vi "VisionNetwork.vi"(8 "error in (no error)":errorcluster) -> (0 "error out":errorcluster)   [LabVIEW 2023]
doc: "Vision Network\n\nInput\n --Error in \n\nOutput\n --Error out"
uses:
  <vilib>/Rock Robotics/WPI/ThirdParty/JAS_Junk/TrajLib/Trajectory_Library.lvlib
  <vilib>/Rock Robotics/Network Tables/NT Write Number.vi
  <vilib>/Rock Robotics/Network Tables/NT Write Boolean.vi
  <vilib>/Rock Robotics/Network Tables/NT Read Number.vi
  Vision/VisionGlobal.vi
  VisionNetworkingGlobal.vi
  <vilib>/Rock Robotics/Network Tables/NT Write Integer.vi
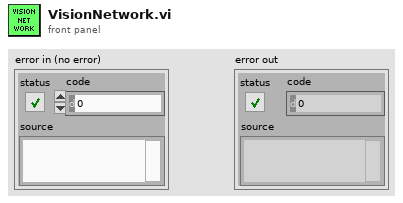
[diagram p1: front panel]
types:
  T1 = typedef "Trajectory_Library.lvlib/POSE2D.ctl" = cluster{"TRANSLATION":T2, "ROTATION":T3}
  T2 = typedef "Trajectory_Library.lvlib/TRANSLATION2D.ctl" = cluster{"X":dbl, "Y":dbl}
  T3 = typedef "Trajectory_Library.lvlib/ROTATION2D.ctl" = cluster{"VALUE":dbl, "COS":dbl, "SIN":dbl}
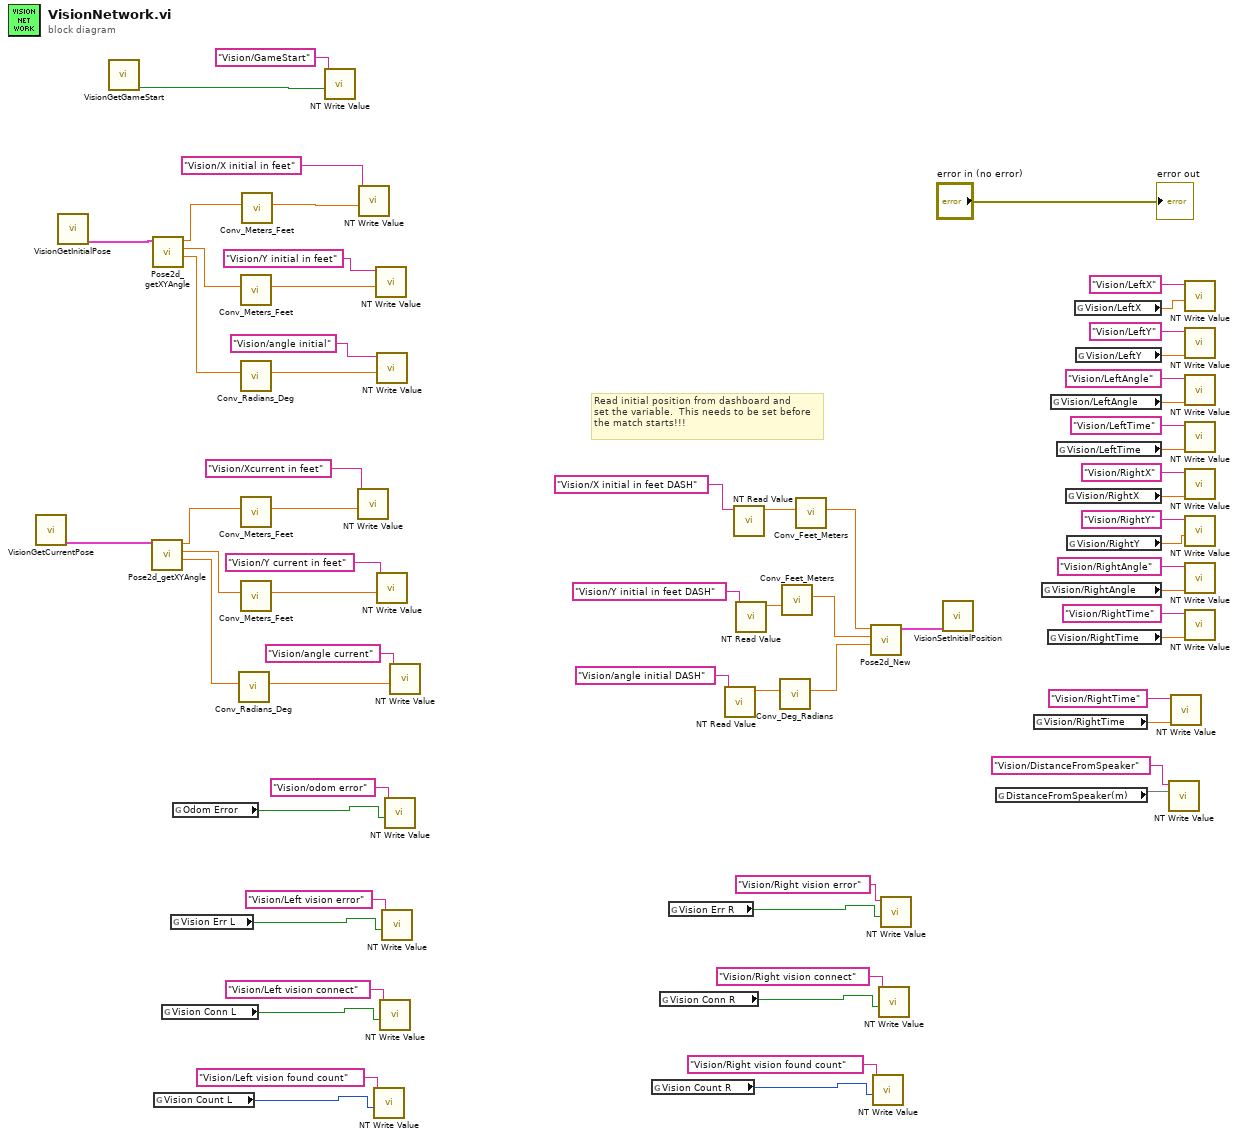
[diagram p0: block diagram]
diagram:
  # "Read initial position from dashboard and\nset the variable.  This needs to be set before\nthe match starts!!!"
  n1 = call "VisionGetCurrentPose.vi"() -> ("Current Pose"=w66:T1)  [unwired: 9 in]
  n2 = call "VisionGetInitialPose.vi"() -> ("InitialPose"=w53:T1)  [unwired: 10 in]
  n3 = call "VisionGetGameStart.vi"() -> ("Game Start"=w52:bool)  [unwired: 11 in]
  n4 = call <vilib>:"Pose2d_getXYAngle.vi"("in POSE"=w66) -> ("Angle"=w65:dbl, "Y"=w64:dbl, "X"=w63:dbl)  [unwired: 8 in]
  n5 = call <vilib>:"Pose2d_getXYAngle.vi"("in POSE"=w53) -> ("Angle"=w59:dbl, "Y"=w58:dbl, "X"=w57:dbl)  [unwired: 8 in]
  n6 = global read "VisionGlobal.vi" "Vision Count L"() -> (w27:i32)
  n7 = global read "VisionGlobal.vi" "Vision Conn L"() -> (w29:bool)
  n8 = global read "VisionGlobal.vi" "Vision Err L"() -> (w31:bool)
  n9 = global read "VisionGlobal.vi" "Odom Error"() -> (w33:bool)
  n10 = call <vilib>:"Conv_Radians_Deg.vi"("Radians"=w65) -> ("Degrees"=w60:dbl)  [unwired: 10 in]
  n11 = call <vilib>:"Conv_Meters_Feet.vi"("Meters"=w58) -> ("Feet"=w55:dbl)  [unwired: 10 in]
  n12 = call <vilib>:"Conv_Radians_Deg.vi"("Radians"=w59) -> ("Degrees"=w54:dbl)  [unwired: 10 in]
  n13 = call <vilib>:"Conv_Meters_Feet.vi"("Meters"=w63) -> ("Feet"=w62:dbl)  [unwired: 10 in]
  n14 = call <vilib>:"Conv_Meters_Feet.vi"("Meters"=w64) -> ("Feet"=w61:dbl)  [unwired: 10 in]
  n15 = call <vilib>:"Conv_Meters_Feet.vi"("Meters"=w57) -> ("Feet"=w56:dbl)  [unwired: 10 in]
  n16 = call-poly <vilib>:"NT Write Value.vi"("value"=w52, "name"="Vision/GameStart") -> ()  [unwired: 9 in, 1 out]
  n17 = call-poly <vilib>:"NT Write Value.vi"("value"=w62, "name"="Vision/Xcurrent in feet") -> ()  [unwired: 9 in, 1 out]
  n18 = call-poly <vilib>:"NT Write Value.vi"("value"=w56, "name"="Vision/X initial in feet") -> ()  [unwired: 9 in, 1 out]
  n19 = call-poly <vilib>:"NT Write Value.vi"("value"=w27, "name"="Vision/Left vision found count") -> ()  [unwired: 9 in, 1 out]
  n20 = call-poly <vilib>:"NT Write Value.vi"("value"=w55, "name"="Vision/Y initial in feet") -> ()  [unwired: 9 in, 1 out]
  n21 = call-poly <vilib>:"NT Write Value.vi"("value"=w54, "name"="Vision/angle initial") -> ()  [unwired: 9 in, 1 out]
  n22 = call-poly <vilib>:"NT Write Value.vi"("value"=w61, "name"="Vision/Y current in feet") -> ()  [unwired: 9 in, 1 out]
  n23 = call-poly <vilib>:"NT Write Value.vi"("value"=w29, "name"="Vision/Left vision connect") -> ()  [unwired: 9 in, 1 out]
  n24 = call-poly <vilib>:"NT Write Value.vi"("value"=w31, "name"="Vision/Left vision error") -> ()  [unwired: 9 in, 1 out]
  n25 = call-poly <vilib>:"NT Write Value.vi"("value"=w33, "name"="Vision/odom error") -> ()  [unwired: 9 in, 1 out]
  n26 = call-poly <vilib>:"NT Write Value.vi"("value"=w60, "name"="Vision/angle current") -> ()  [unwired: 9 in, 1 out]
  n27 = global read "VisionGlobal.vi" "Vision Count R"() -> (w22:i32)
  n28 = global read "VisionGlobal.vi" "Vision Conn R"() -> (w24:bool)
  n29 = global read "VisionGlobal.vi" "Vision Err R"() -> (w26:bool)
  n30 = call-poly <vilib>:"NT Read Value.vi"("name"="Vision/angle initial DASH") -> ("value"=w39:dbl)  [unwired: 8 in, 2 out]
  n31 = call-poly <vilib>:"NT Read Value.vi"("name"="Vision/X initial in feet DASH") -> ("value"=w42:dbl)  [unwired: 8 in, 2 out]
  n32 = call-poly <vilib>:"NT Read Value.vi"("name"="Vision/Y initial in feet DASH") -> ("value"=w41:dbl)  [unwired: 8 in, 2 out]
  n33 = call <vilib>:"Conv_Deg_Radians.vi"("Degress"=w39) -> ("Radians"=w38:dbl)  [unwired: 10 in]
  n34 = call <vilib>:"Conv_Feet_Meters.vi"("Feet"=w41) -> ("Meters"=w40:dbl)  [unwired: 10 in]
  n35 = call <vilib>:"Conv_Feet_Meters.vi"("Feet"=w42) -> ("Meters"=w43:dbl)  [unwired: 10 in]
  n36 = call <vilib>:"Pose2d_New.vi"("Heading"=w38, "Y"=w40, "X"=w43) -> ("out POSe"=w44:T1)  [unwired: 8 in]
  n37 = call-poly <vilib>:"NT Write Value.vi"("value"=w22, "name"="Vision/Right vision found count") -> ()  [unwired: 9 in, 1 out]
  n38 = call-poly <vilib>:"NT Write Value.vi"("value"=w24, "name"="Vision/Right vision connect") -> ()  [unwired: 9 in, 1 out]
  n39 = call-poly <vilib>:"NT Write Value.vi"("value"=w26, "name"="Vision/Right vision error") -> ()  [unwired: 9 in, 1 out]
  n40 = call "VisionSetInitialPosition.vi"("InitialPose"=w44) -> ()  [unwired: 11 in]
  n41 = global read "VisionGlobal.vi" "DistanceFromSpeaker(m)"() -> (w2)
  n42 = global read "VisionNetworkingGlobal.vi" "Vision/RightTime"() -> (w3:dbl)
  n43 = global read "VisionNetworkingGlobal.vi" "Vision/RightAngle"() -> (w7:dbl)
  n44 = global read "VisionNetworkingGlobal.vi" "Vision/RightTime"() -> (w5:dbl)
  n45 = global read "VisionNetworkingGlobal.vi" "Vision/LeftAngle"() -> (w15:dbl)
  n46 = global read "VisionNetworkingGlobal.vi" "Vision/LeftTime"() -> (w13:dbl)
  n47 = global read "VisionNetworkingGlobal.vi" "Vision/RightX"() -> (w11:dbl)
  n48 = global read "VisionNetworkingGlobal.vi" "Vision/RightY"() -> (w9:dbl)
  n49 = global read "VisionNetworkingGlobal.vi" "Vision/LeftX"() -> (w19:dbl)
  n50 = global read "VisionNetworkingGlobal.vi" "Vision/LeftY"() -> (w17:dbl)
  n51 = call-poly <vilib>:"NT Write Value.vi"("value"=w2, "name"="Vision/DistanceFromSpeaker") -> ()  [unwired: 9 in, 1 out]
  n52 = call-poly <vilib>:"NT Write Value.vi"("value"=w3, "name"="Vision/RightTime") -> ()  [unwired: 9 in, 1 out]
  n53 = call-poly <vilib>:"NT Write Value.vi"("value"=w19, "name"="Vision/LeftX") -> ()  [unwired: 9 in, 1 out]
  n54 = call-poly <vilib>:"NT Write Value.vi"("value"=w17, "name"="Vision/LeftY") -> ()  [unwired: 9 in, 1 out]
  n55 = call-poly <vilib>:"NT Write Value.vi"("value"=w15, "name"="Vision/LeftAngle") -> ()  [unwired: 9 in, 1 out]
  n56 = call-poly <vilib>:"NT Write Value.vi"("value"=w13, "name"="Vision/LeftTime") -> ()  [unwired: 9 in, 1 out]
  n57 = call-poly <vilib>:"NT Write Value.vi"("value"=w11, "name"="Vision/RightX") -> ()  [unwired: 9 in, 1 out]
  n58 = call-poly <vilib>:"NT Write Value.vi"("value"=w9, "name"="Vision/RightY") -> ()  [unwired: 9 in, 1 out]
  n59 = call-poly <vilib>:"NT Write Value.vi"("value"=w7, "name"="Vision/RightAngle") -> ()  [unwired: 9 in, 1 out]
  n60 = call-poly <vilib>:"NT Write Value.vi"("value"=w5, "name"="Vision/RightTime") -> ()  [unwired: 9 in, 1 out]
  "error out" <- "error in (no error)"
